vi "Merge Patch ATTEMPT 2.vi"(4 "null means delete (T)":bool=TRUE, 6 "Item Name":string, 7 "Object (or Item) Path":string, 8 "error in (no error)":errorcluster, 9 "JSON Patch":string, 10 "Object Offset":i32, 11 "JSON in":string="{}") -> (0 "error out":errorcluster, 3 "<JSON>":string)   [LabVIEW 2015, in "JSONtext.lvlib"]
doc: "Insert JSON item at the Path specified."
uses:
  JSONtext.lvlib
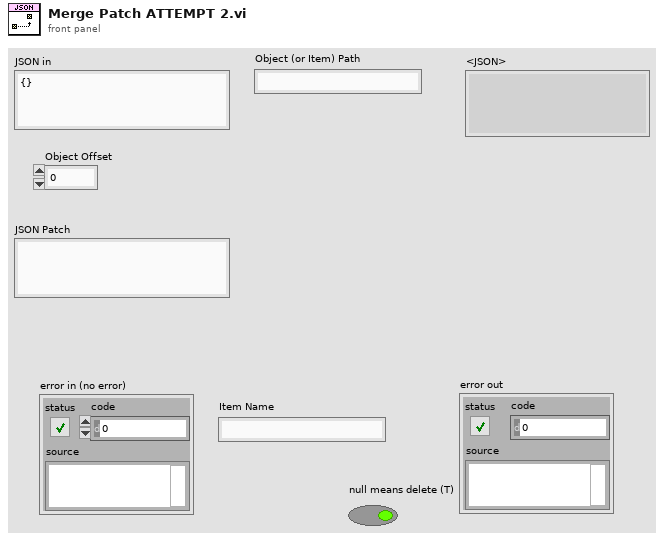
[diagram p1: front panel]
types:
  T1 = typedef "JSONtext.lvlib/Found Items.ctl" = cluster{"Item offset":i32, "Offset past Item":i32, "Name offset":i32, "Offset past Name":i32, "Found":bool, "Item Type":T2, "Item Index":i32}
  T2 = typedef "JSONtext.lvlib/Parsing State.ctl" = enum16{"Parser Error", "Object", "Array", "String", "Number/Other", "Leading Whitespace", "Object end", "Array end", "Value end"}
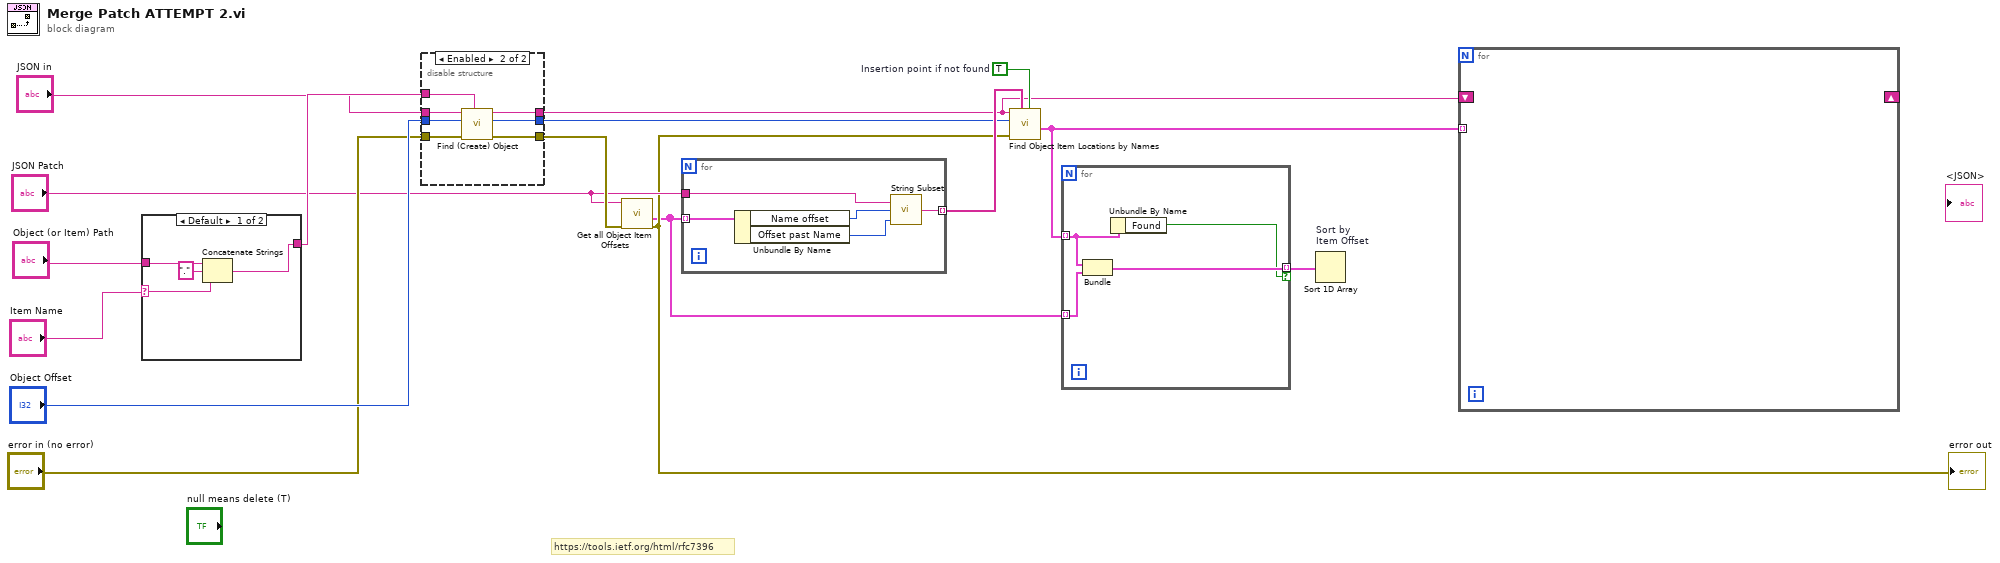
[diagram p0: block diagram]
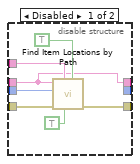
[diagram p2: hidden frame]
diagram:
  w8 = TRUE  # Insertion point if not found
  # "https://tools.ietf.org/html/rfc7396"
  n1 = case shown="Default" "Item Name" {
    selector: "Item Name" -> [w17 _]
    tunnel: "Object (or Item) Path" -> [w20 w21]
    tunnel: [w18 w21] -> w11
    frame Default {
      n2 = Concatenate Strings(w20, "." ("string"), w17) -> (w18:string)
    }
    frame "" {
    }
  }
  n3 = disable-structure shown="Enabled" {
    disable-tunnel: "Object Offset" -> [w28 w32]
    disable-tunnel: "error in (no error)" -> [w25 w33]
    disable-tunnel: [w24 w31] -> w12
    disable-tunnel: w11 -> [w23 w34]
    disable-tunnel: "JSON in" -> [w22 w35]
    disable-tunnel: [w22 w30] -> w4
    disable-tunnel: [_ w29] -> w6
    frame Disabled {
      n4 = call "Find Item Locations by Path.vi"("Insertion point if not found"=TRUE, "Only return first found"=TRUE, "Path"=w23, "error in (no error)"=w25, "Object Offset"=w28, "JSON"=w22) -> ("error out"=w24:errorcluster)  [unwired: 4 in, 1 out]
    }
    frame Enabled {
      n5 = call "Find (Create) Object.vi"("Object Path"=w34, "error in (no error)"=w33, "Starting Offset"=w32, "JSON"=w35) -> ("error out"=w31:errorcluster, "Object offset"=w29:i32, "<JSON>"=w30:string)  [unwired: 5 in]
    }
  }
  n6 = call "Get all Object Item Offsets.vi"("error in (no error)"=w12, "JSON"="JSON Patch") -> ("error out"=w5:errorcluster, "Items"=w2:T1[])  [unwired: 7 in, 1 out]
  "error out" <- w5
  n7 = for {
    tunnel: w2 -> [w40] mode=indexing
    tunnel: "JSON Patch" -> [w37]
    tunnel: [w36] -> w7 mode=indexing
    n8 = Unbundle By Name(w40) -> ("Name offset"=w39:i32, "Offset past Name"=w38:i32)
    n9 = call "String Subset.vi"("Offset past End"=w38, "Start offset"=w39, "JSON"=w37) -> ("substring"=w36:string)  [unwired: 2 in]
  }
  n10 = call "Find Object Item Locations by Names.vi"("Insertion point if not found"=w8, "Item Names <JSON>"=w7, "error in (no error)"=w5, "Object Offset"=w6, "JSON"=w4) -> ("Items"=w3:T1[])  [unwired: 5 in, 1 out]
  n11 = for {
    tunnel: w3 -> [w42] mode=indexing
    tunnel: w2 -> [w44] mode=indexing
    tunnel: [w43] -> w1 mode=indexing if=w41
    n12 = Bundle("Item"=w42, w44) -> (w43:cluster{"Item":T1, T1})  [unwired: 1 in]
    n13 = Unbundle By Name(w42) -> ("Found"=w41:bool)
  }
  n14 = Sort 1D Array "Sort by \nItem Offset"(array=w1) -> ()  [unwired: 1 out]
  n15 = for {
    tunnel: w3 -> [_] mode=indexing
    shift-right: _ -> [_]
    shift-left: w4 -> [_]
  }
